vi "CSGaussmeter.setUpper.vi"(0 "i ref in":refnum<vi>, 7 "upper":dbl, 9 "Unit":T1, 11 "error in (no error)":errorcluster) -> (4 "i ref out":refnum<vi>, 15 "error out":errorcluster)   [LabVIEW 2014, in "CSGaussmeter.lvlib"]
doc: "Dieses VI setzt die Obergrenze für die Limit-Funktion\n\n\nThis VI sets the upper limit for the limit function"
uses:
  CSGaussmeter.lvlib
  instr.lib/FH_55/TypeDef/Unit2.ctl
  CS_Core/CSObj/CSObj.lvlib
  CSlibraries/UtilityLib/UtilityLib.lvlib
  instr.lib/FH_55/FH 55.lvlib
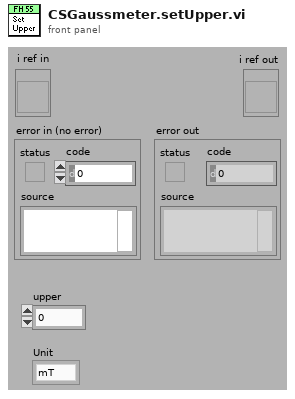
[diagram p1: front panel]
types:
  T1 = typedef "FH 55.lvlib/Unit2.ctl" = enum16{"mT", "G", "kA/m"}
  T2 = typedef "CSGaussmeter.lvlib/CSGaussmeter.i attribute.ctl" = cluster{"Name":string, "VISA Resource Name":refnum<visa-resource-name>, "actValues":cluster{" Limit":bool, "Unit ":T3, "Temp_Unit":T4, "Max":T5, " Filter":bool, " Peak":bool, " Auto_Range":bool, "Range":T6, " Rel":bool, " CTemp":bool, " CField":bool, "AC_DC ":bool, "Set_lower":cluster{"Numeric":dbl, "Cancel Button":bool, "Unit":T1}, "Set_upper":cluster{"Numeric":dbl, "Cancel Button":bool, "Unit":T1}, "Set_Rel":cluster{"Numeric":dbl, "Cancel Button":bool, "Unit":T1}, "Zero":bool, " Local":bool, "Reset":bool, " Init":bool}, "FH 55 Gauss-/Teslameter":T7, "MAX_Value":T8, "MIN_Value":T8, "Rel_Value":T8, "Array ":string[], "LIMU":dbl, " LIML":dbl, "Messwerte 2":string, "Messwerte ":cluster{"Numeric":i32, "OK Button":bool}, "serviceID":cluster{"Current ID":i32, "Unit ID":i32, "Temp ID":i32, "Name ID \n":i32, "Visa ID ":i32}, "setValues ":cluster{" Limit":bool, "Unit ":T3, "Temp_Unit":T4, "Max":T5, " Filter":bool, " Peak":bool, " Auto_Range":bool, "Range":T6, " Rel":bool, " CTemp":bool, " CField":bool, "AC_DC ":bool, "Set_lower":cluster{"Numeric":dbl, "Cancel Button":bool, "Unit":T1}, "Set_upper":cluster{"Numeric":dbl, "Cancel Button":bool, "Unit":T1}, "Set_Rel":cluster{"Numeric":dbl, "Cancel Button":bool, "Unit":T1}, "Zero":bool, " Local":bool, "Reset":bool, " Init":bool}}
  T3 = typedef "FH 55.lvlib/Unit.ctl" = enum16{"T", "G", "A/m"}
  T4 = typedef "FH 55.lvlib/Temp_Unit.ctl" = enum16{"Temp off", "Celsius", "Fahrenheit"}
  T5 = typedef "FH 55.lvlib/Max.ctl" = enum16{"MAX off", "Show MAX", "MAX/MIN"}
  T6 = typedef "FH 55.lvlib/Range.ctl" = enum16{"1", "2", "3", "4", "5", "6", "7"}
  T7 = typedef "FH 55.lvlib/Display.ctl" = cluster{"current value":string, "Limit":string, "Remote":string, "function ":string, "Cluster":cluster{"AC/DC":string, "Auto":string, "Filter":string, "Range":string, "Rel":string, "Peak":string}}
  T8 = typedef "FH 55.lvlib/Value_String.ctl" = cluster{"Numeric":dbl, "String":string}
  T9 = cluster{"Numeric":dbl, "Cancel Button":bool, "Unit":T1}
  T10 = cluster{"VISA Resource Name":refnum<visa-resource-name>}
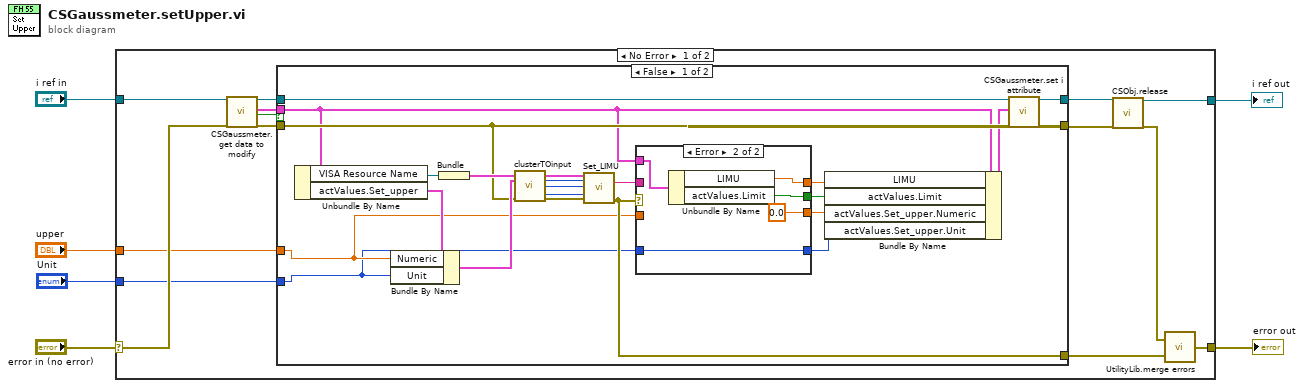
[diagram p0: block diagram]
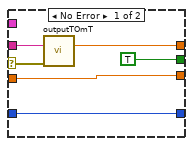
[diagram p2: hidden frame]
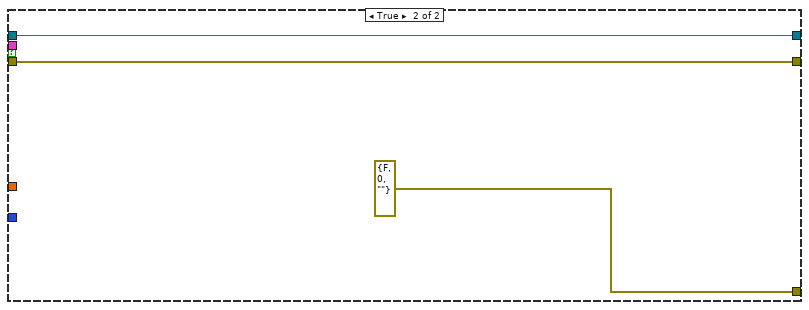
[diagram p3: hidden frame]
diagram:
  n1 = case shown="No Error" "error in (no error)" {
    selector: "error in (no error)" -> [w15 w57]
    tunnel: [w16 w57] -> w3
    tunnel: "i ref in" -> [w14 w58]
    tunnel: [w7 w58] -> w4
    tunnel: "upper" -> [w8 _]
    tunnel: "Unit" -> [w9 _]
    frame No Error {
      n2 = call "CSGaussmeter.get data to modify.vi"("i ref in"=w14, "error in (no error)"=w15) -> ("i ref out"=w13:refnum<vi>, "i attribute"=w12:T2, "timed out"=w11:bool, "error out"=w10:errorcluster)  [unwired: 14 in]
      n3 = case shown="False" w11 {
        tunnel: w13 -> [w41 w55]
        tunnel: w10 -> [w29 w56]
        tunnel: w12 -> [w21 _]
        tunnel: [w28 w56] -> w18
        tunnel: [w40 w55] -> w20
        tunnel: [w26 errorcluster {"status"=FALSE, "code"=0, "source"=""} ("error out")] -> w17
        tunnel: w9 -> [w23 _]
        tunnel: w8 -> [w25 _]
        frame False {
          n4 = Unbundle By Name(w21) -> ("VISA Resource Name"=w42:refnum<visa-resource-name>, "actValues.Set_upper"=w27:T9)
          n5 = Bundle By Name(cluster=w27, "Numeric"=w25, "Unit"=w23) -> (w33:T9)
          n6 = Bundle("VISA Resource Name"=w42) -> (w39:T10)  [unwired: 1 in]
          n7 = call "clusterTOinput.vi"("Set_Rel"=w33, "error in (no error)"=w29) -> ("Range"=w30:T6, "Numeric"=w31:i32, "Unit"=w32:T3, "error out"=w34:errorcluster)  [unwired: 10 in]
          n8 = call "Set_LIMU.vi"("VisaCluster"=w39, "Range"=w30, "Ziffern"=w31, "Unit"=w32, "error in (no error)"=w34) -> ("Answer"=w38:string, "error out"=w26:errorcluster)  [unwired: 8 in, 1 out]
          n9 = case shown="Error" w26 {
            selector: w26 -> [w45 _]
            tunnel: w38 -> [w48 _]
            tunnel: [TRUE ("actValues.Limit") w50] -> w36
            tunnel: [w46 w49] -> w35
            tunnel: w25 -> [w44 _]
            tunnel: [w44 0.0 ("Numeric")] -> w24
            tunnel: [w43 w53] -> w22
            tunnel: w23 -> [w43 w53]
            tunnel: w21 -> [_ w51]
            frame No Error {
              n10 = call "outputTOmT.vi"("Input"=w48, "error in (no error)"=w45) -> ("Numeric"=w46:dbl)  [unwired: 12 in, 1 out]
            }
            frame Error {
              n11 = Unbundle By Name(w51) -> ("LIMU"=w49:dbl, "actValues.Limit"=w50:bool)
            }
          }
          n12 = Bundle By Name(cluster=w21, "LIMU"=w35, "actValues.Limit"=w36, "actValues.Set_upper.Numeric"=w24, "actValues.Set_upper.Unit"=w22) -> (w37:T2)
          n13 = call "CSGaussmeter.set i attribute.vi"("i ref in"=w41, "i attribute"=w37, "error in (no error)"=w29) -> ("i ref out"=w40:refnum<vi>, "error out"=w28:errorcluster)  [unwired: 15 in]
        }
        frame True {
        }
      }
      n14 = call "CSObj.release.vi"("i ref in"=w20, "error in (no error)"=w18) -> ("i ref out"=w7:refnum<vi>, "error out"=w19:errorcluster)  [unwired: 16 in]
      n15 = call "UtilityLib.merge errors.vi"("error2 (no error)"=w17, "error1 (no error)"=w19) -> ("error out"=w16:errorcluster)
    }
    frame Error {
    }
  }
  "i ref out" <- w4
  "error out" <- w3
